vi "READ - Multiples Files.vi"(0 "reference in":refnum<class "TDMS.lvclass">, 5 "error in (no error)":errorcluster, 7 "File List":path[](array[path]), 9 "Valid T0":bool) -> (14 "reference out":refnum<class "TDMS.lvclass">, 19 "error out":errorcluster)   [LabVIEW 2022 SP3, in "TDMS.lvclass"]
uses:
  TDMS.lvclass
  API/GSwFormDSP_class/functions/Attribute List.ctl
  API/GSwFormDSP_class/GSwFormDSP.lvclass
  API/Generic Utilities_class/Generic Utilities.lvclass
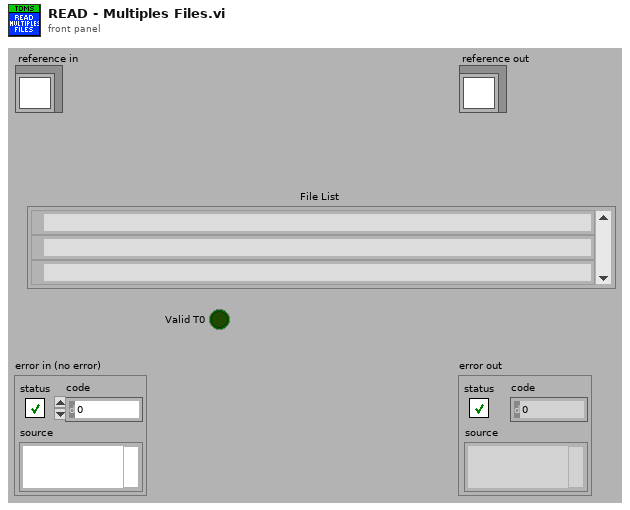
[diagram p1: front panel]
types:
  T1 = typedef "GSwFormDSP.lvclass/Attribute List.ctl" = string
  T2 = typedef "TDMS.lvclass/ObjectAttributesRef.ctl" = refnum<data-value>
  T3 = typedef "TDMS.lvclass/ObjectAttributes.ctl" = cluster{"Time Data":refnum<class "GSwFormDSP.lvclass">, "New Time Data Obj?":bool}
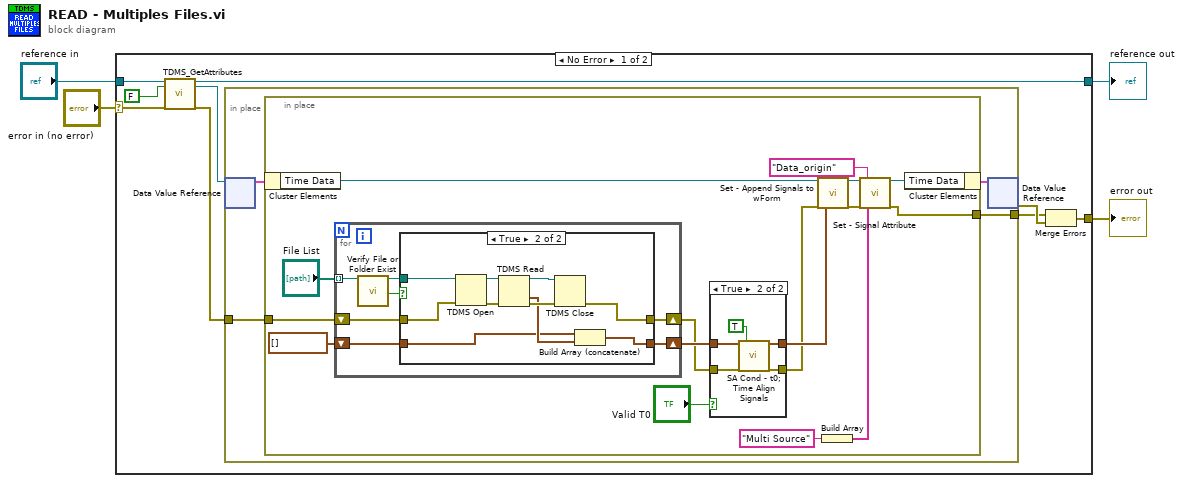
[diagram p0: block diagram]
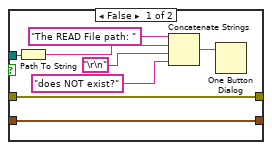
[diagram p3: hidden frame]
diagram:
  n1 = case shown="No Error" "error in (no error)" {
    selector: "error in (no error)" -> [w8 w67]
    tunnel: [w13 w67] -> w3
    tunnel: [w7 w66] -> w1
    tunnel: "reference in" -> [w10 w66]
    frame No Error {
      n2 = call "TDMS_GetAttributes.vi"("reference in"=w10, "return data? (T)"=FALSE, "error in (no error)"=w8) -> ("reference out"=w7:refnum<class "TDMS.lvclass">, "attributes ref"=w6:T2, "error out"=w5:errorcluster)  [unwired: 13 in, 1 out]
      n3 = in-place {
        in-place-border: [w14] -> w11
        in-place-border: w5 -> [w15]
        n4 = in-place-dvr #1(w6) -> (w16:T3)  [unwired: 1 out]
        n5 = in-place {
          in-place-border: w15 -> [w33]
          in-place-border: [w26] -> w14
          n6 = in-place-cluster #2(w16) -> ("Time Data"=w25:refnum<class "GSwFormDSP.lvclass">)
          n7 = for {
            tunnel: "File List" -> [w43] mode=indexing
            shift-right: [w42] -> w21
            shift-left: waveform(dbl)[] [] -> [w41]
            shift-right: [w44] -> w19
            shift-left: w33 -> [w45]
            n8 = call "Verify File or Folder Exist.vi"("path"=w43) -> ("dup path"=w47:path, "file or folder exists?"=w46:bool)  [unwired: 16 in, 1 out]
            n9 = case shown="True" w46 {
              tunnel: w47 -> [w54 w65]
              tunnel: w45 -> [w55 w64]
              tunnel: [w55 w59] -> w44
              tunnel: [w48 w57] -> w42
              tunnel: w41 -> [w48 w56]
              frame False {
                n10 = Path To String(path=w54) -> (string=w52:string)
                n11 = Concatenate Strings("The READ File path: ", w52, "\r\n", "does NOT exist?") -> (w49:string)
                n12 = One Button Dialog(message=w49) -> ()  [unwired: 1 in, 1 out]
              }
              frame True {
                n13 = TDMS Open(8:w64, 11:w65) -> (0:w63:errorcluster, 3:w62:refnum<k34>)  [unwired: 5 in]
                n14 = TDMS Read(0:w62, 11:w63) -> (4:w60:refnum<k34>, 10:w58:waveform(dbl)[], 15:w61:errorcluster)  [unwired: 6 in, 3 out]
                n15 = TDMS Close(8:w61, 11:w60) -> (0:w59:errorcluster)  [unwired: 1 out]
                n16 = Build Array (concatenate)(w56, w58) -> (w57:waveform(dbl)[])
              }
            }
          }
          n17 = case shown="True" "Valid T0" {
            tunnel: w21 -> [w34 w40]
            tunnel: [w34 w39] -> w20
            tunnel: w19 -> [w35 w37]
            tunnel: [w35 w36] -> w18
            frame False {
            }
            frame True {
              n18 = call "SA Cond - t0; Time Align Signals.vi"("Signal IN"=w40, "error in (no error)"=w37, "Anotate Signal Name"=TRUE) -> ("Signal OUT"=w39:waveform(dbl)[], "error out"=w36:errorcluster)  [unwired: 15 in]
            }
          }
          n19 = call "Set - Append Signals to wForm.vi"("reference in"=w25, "error in (no error)"=w18, "New Signals"=w20) -> ("reference out"=w31:refnum<class "GSwFormDSP.lvclass">, "error out"=w30:errorcluster)  [unwired: 15 in]
          n20 = Build Array("Multi Source") -> (w29:string[])
          n21 = call-dynamic "Set - Signal Attribute.vi"("reference in"=w31, "error in (no error)"=w30, "wForm Attributes"=T1 "Data_origin", "Attribute"=w29) -> ("reference in"=w24:refnum<class "GSwFormDSP.lvclass">, "error out"=w26:errorcluster)  [unwired: 14 in]
          n22 = in-place-cluster #2("Time Data"=w24) -> (w17:T3)
        }
        n23 = in-place-dvr #1(w17) -> (w12:errorcluster)  [unwired: 1 out]
      }
      n24 = Merge Errors(w11, w12) -> (w13:errorcluster)
    }
    frame Error {
    }
  }
  "error out" <- w3
  "reference out" <- w1
